vi "S2C_5190CR_Proc_Status.vi"(8 "Error In":errorcluster) -> (0 "Error Out":errorcluster, 3 "Response":string)   [LabVIEW 2015]
uses:
  S2C_5190CR_Proc_Globals.vi
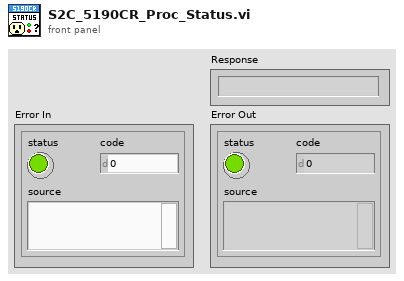
[diagram p1: front panel]
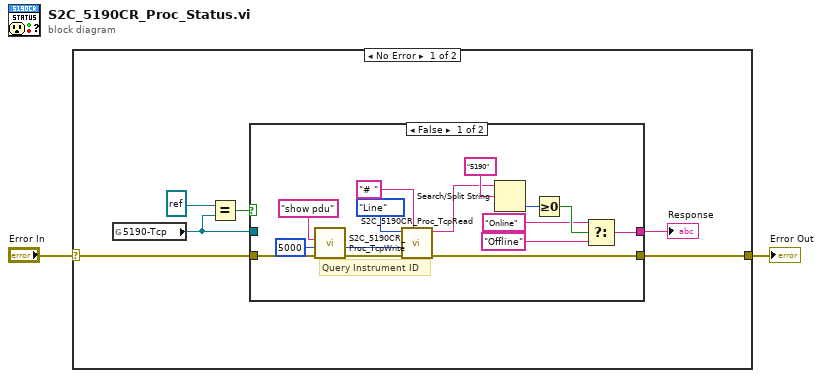
[diagram p0: block diagram]
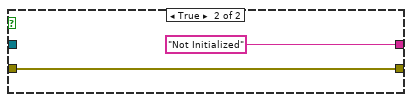
[diagram p2: hidden frame]
diagram:
  n1 = case shown="No Error" "Error In" {
    selector: "Error In" -> [w8 w25]
    tunnel: [w7 w25] -> w1
    frame No Error {
      n2 = global read "S2C_5190CR_Proc_Globals.vi" "5190-Tcp"() -> (w3:refnum<k5>)
      n3 = Equal?(x=refnum<k5> refnum ("5190-Tcp"), y=w3) -> (x = y?=w5:bool)
      n4 = case shown="False" w5 {
        tunnel: w8 -> [w16 w24]
        tunnel: w3 -> [_ _]
        tunnel: [w13 w24] -> w7
        tunnel: [w17 "Not Initialized" ("f")] -> w6
        frame False {
          w10 = 5000 ("Timeout(ms)")
          # "Query Instrument ID"
          n5 = call "S2C_5190CR_Proc_TcpWrite.vi"("Error In"=w16, "Timeout(ms)"=w10, "Data"="show pdu" ("write buffer")) -> ("Error Out"=w14:errorcluster)  [unwired: 8 in]
          n6 = call "S2C_5190CR_Proc_TcpRead.vi"("Line Seperator"="# " ("line separator"), "Error In"=w14, "Timeout(ms)"=w10, "Read Mode"=enum16{"Normal", "Line"}."Line") -> ("Error Out"=w13:errorcluster, "Data"=w12:string)  [unwired: 6 in]
          n7 = Search/Split String(string=w12, search string/char (-)="5190") -> (offset of match=w21:i32)  [unwired: 1 in, 2 out]
          n8 = Greater Or Equal To 0?(x=w21) -> (x >= 0?=w20:bool)
          n9 = Select(t="Online", s=w20, f="Offline") -> (s? t:f=w17:string)
        }
        frame True {
        }
      }
      "Response" <- w6
    }
    frame Error {
    }
  }
  "Error Out" <- w1
